vi "HapticIO_11.vi"() -> ()   [LabVIEW 2017]
uses:
  <userlib>/PositionDLL/PositionDLL.lvlib
panel:
  out "FW":dbl
  out "VY":dbl
  out "VZ":dbl
  out "VX":dbl
  in  "Drag":dbl=1.0
  in  "STOP":bool
  in  "START":bool
  out "Fy":dbl
  out "Fz":dbl
  out "phi":dbl
  out "psi":dbl
  out "Fx":dbl
  out "theta":dbl
  out "x":dbl
  out "y":dbl
  out "z":dbl
  in  "Sensitivity":dbl=3.5
  out "Clicks":dbl
  out "Scope":dbl
  out "FH":dbl
  out "XI":dbl
  out "ZI":dbl
  # "Sample Window"
  # "Position"
  # "Force"
  # "Angles"
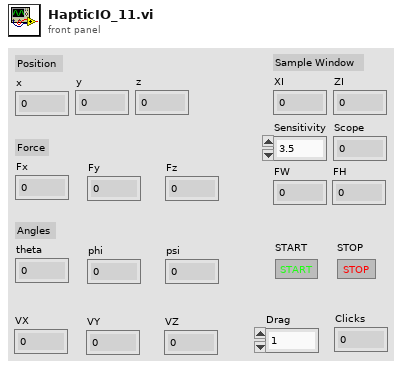
[diagram p1: front panel]
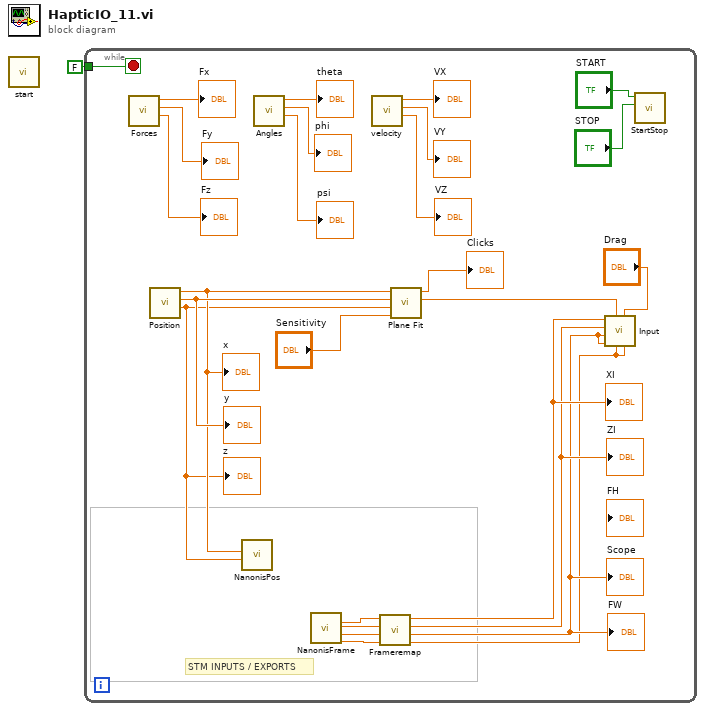
[diagram p0: block diagram]
diagram:
  n1 = call <userlib>:"start.vi"() -> ()  [unwired: 11 in, 1 out]
  n2 = while {
    tunnel: FALSE -> [w16]
    stop <- w16 stop-if-true
    # "STM INPUTS / EXPORTS"
    n3 = call <userlib>:"Forces.vi"() -> ("Fz"=→"Fz":dbl, "Fy"=→"Fy":dbl, "Fx"=→"Fx":dbl)  [unwired: 9 in]
    n4 = call <userlib>:"Position.vi"() -> ("Z"=w9:dbl, "Y"=w23:dbl, "X"=w10:dbl)  [unwired: 9 in]
    "x" <- w10
    "y" <- w23
    "z" <- w9
    n5 = call <userlib>:"NanonisPos.vi"("z"=w9, "x"=w10) -> ()  [unwired: 9 in, 1 out]
    n6 = call <userlib>:"Angles.vi"() -> ("psi"=→"psi":dbl, "phi"=→"phi":dbl, "theta"=→"theta":dbl)  [unwired: 9 in]
    n7 = call <userlib>:"NanonisFrame.vi"() -> ("FO X"=w8:dbl, "FO Z"=w7:dbl, "FW"=w6:dbl, "FH"=w5:dbl)  [unwired: 11 in, 1 out]
    n8 = call <userlib>:"velocity.vi"() -> ("VZ"=→"VZ":dbl, "VY"=→"VY":dbl, "VX"=→"VX":dbl)  [unwired: 9 in]
    n9 = call "Frameremap.vi"("FH"=w5, "FW"=w6, "FO Z"=w7, "FO X"=w8) -> ("FH"=w2:dbl, "FW"=w3:dbl, "Z Origin"=w18:dbl, "X Origin"=w19:dbl)  [unwired: 4 in]
    "Scope" <- w3
    "XI" <- w19
    "ZI" <- w18
    "FW" <- w3
    n10 = call <userlib>:"Plane Fit.vi"("Sensitivity"="Sensitivity", "Z"=w9, "Y"=w23, "X"=w10) -> ("Output"=w20:dbl, "Clicks"=→"Clicks":dbl)  [unwired: 6 in]
    n11 = call <userlib>:"Input.vi"("Scopez"=w2, "Drag"="Drag", "FH"=w2, "Signal in"=w20, "FW"=w3, "Scopex"=w3, "Z origin"=w18, "X origin"=w19) -> ()  [unwired: 4 in]
    n12 = call <userlib>:"StartStop.vi"("STOP"="STOP", "START"="START") -> ()  [unwired: 10 in]
  }
